vi "Get Transfer Configurations.vi"(8 "error in (no error)":errorcluster, 11 "Group Configuration in":refnum<class "Group Configuration.lvclass">) -> (0 "error out":errorcluster, 2 "Transfer Configurations":refnum<class "Transfer Configuration.lvclass">[](array[class]), 3 "Group Configuration out":refnum<class "Group Configuration.lvclass">)   [LabVIEW 2017, in "DSF Core.lvlib" / "Group Configuration.lvclass"]
uses:
  Group Configuration.lvclass
  Transfer/Transfer Configuration.lvclass
  Group Configuration.lvclass/Group Configuration.ctl
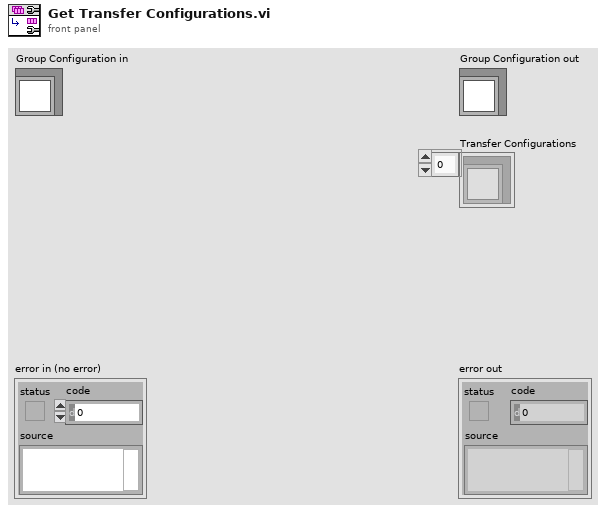
[diagram p1: front panel]
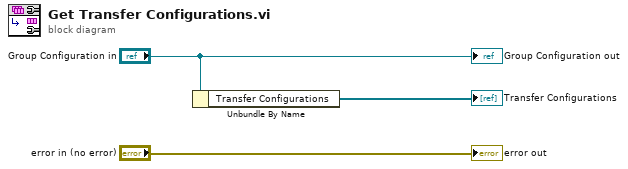
[diagram p0: block diagram]
diagram:
  n1 = Unbundle By Name("Group Configuration in") -> ("Transfer Configurations"=→"Transfer Configurations":refnum<class "Transfer Configuration.lvclass">[])
  "error out" <- "error in (no error)"
  "Group Configuration out" <- "Group Configuration in"
